vi "Mux_development_test.vi"   [LabVIEW 2018]
uses:
  InstrControl/Switching/Switching.lvclass
  InstrControl/InstrControl.lvclass
types:
  T1 = enum16{"Reset", "Ground", "Striptest SMU", "Striptest LCR", "IV", "CV", "Interstrip Cap", "Interstrip Res"}
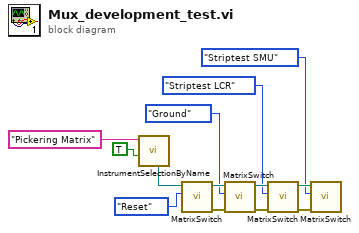
[diagram p0: block diagram]
diagram:
  n1 = call "InstrumentSelectionByName.vi"("Verify GPIB address"=TRUE, "Instrument name IN"="Pickering Matrix") -> ("Switching"=w11:refnum<class "Switching.lvclass">)  [unwired: 4 in, 5 out]
  n2 = call-dynamic "MatrixSwitch.vi"("Action"=T1."Reset", "Switching in"=w11) -> ("error out"=w9:errorcluster, "Switching out"=w8:refnum<class "Switching.lvclass">)  [unwired: 7 in, 1 out]
  n3 = call-dynamic "MatrixSwitch.vi"("error in (no error)"=w9, "Action"=T1."Ground", "Switching in"=w8) -> ("error out"=w7:errorcluster, "Switching out"=w6:refnum<class "Switching.lvclass">)  [unwired: 6 in, 1 out]
  n4 = call-dynamic "MatrixSwitch.vi"("error in (no error)"=w7, "Action"=T1."Striptest LCR", "Switching in"=w6) -> ("error out"=w3:errorcluster, "Switching out"=w2:refnum<class "Switching.lvclass">)  [unwired: 6 in, 1 out]
  n5 = call-dynamic "MatrixSwitch.vi"("error in (no error)"=w3, "Action"=T1."Striptest SMU", "Switching in"=w2) -> ()  [unwired: 6 in, 3 out]
